vi "Start Actor.vi"(8 "error in (no error)":errorcluster, 10 "Initial Music Library":refnum<class "MusicLibrary.lvclass">, 11 "MusicManagerActor In":refnum<class "MusicManagerActor.lvclass">) -> (0 "error out":errorcluster, 3 "MusicManagerActor Out":refnum<class "MusicManagerActor.lvclass">)   [LabVIEW 2015, in "MusicManagerActor.lvlib" / "MusicManagerActor.lvclass"]
uses:
  MusicManagerActor.lvclass
  file/MusicElement/MusicElementLibrary/MusicLibrary/MusicLibrary.lvclass
  MusicManagerActor.lvclass/MusicManagerActor.ctl
  <vilib>/ActorFramework/Actor/Actor.lvclass
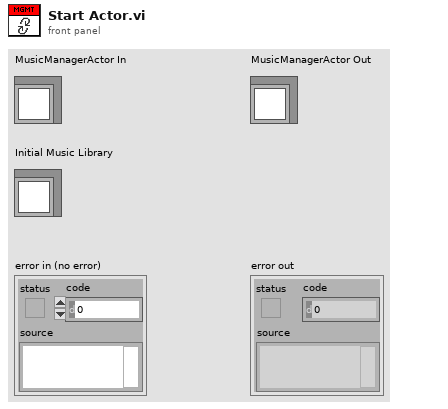
[diagram p1: front panel]
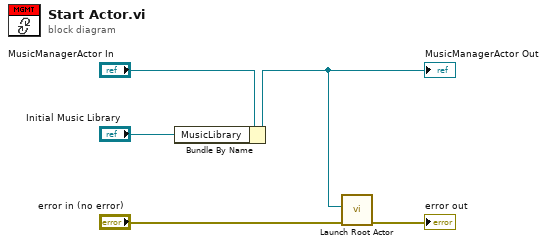
[diagram p0: block diagram]
diagram:
  n1 = Bundle By Name(cluster="MusicManagerActor In", "MusicLibrary"="Initial Music Library") -> (w2:refnum<class "MusicManagerActor.lvclass">)
  "MusicManagerActor Out" <- w2
  n2 = call <vilib>:"Launch Root Actor.vi"("error in (no error)"="error in (no error)", "Actor"=w2) -> ("error out"=→"error out":errorcluster)  [unwired: 8 in, 1 out]
